vi "MirrorSlidePan.vi"(8 "error in (no error)":errorcluster caption="entrée d'erreur (pas d'erreur)", 11 "ESP301.lvclass":refnum<class "ESP301.lvclass">) -> (0 "error out":errorcluster caption="sortie d'erreur", 3 "ESP301.lvclass Out":refnum<class "ESP301.lvclass">)   [LabVIEW 2019, in "ESP301.lvclass"]
uses:
  ESP301.lvclass
  C:/Programmes Labview/LabscanV1A/DevicesClass/BaseDevice/BaseDevice.lvclass
  ESP301.lvclass/ESP301.ctl
  BaseDevice/ClassQueueMess.ctl
  BaseDevice/Accessor/GetClassEvent.vi
panel:
  out "ESP_pos":refnum<vi>
  out "APDs":bool
  in  "Con/Disc.":bool
  out "Homed":bool
  in  "Enable":bool
  in  "Home":bool caption="MiseAJour"
  out "Moving":bool
  out "Axis Model":string
  out "Valid Ref":bool
  out "BKD Lim":bool
  out "FWD Lim":bool
  in  "Axis 1":u8(ring)=1 items=["1"=1, "2"=2, "3"=3]
  out "ActPos":dbl=60.0 caption="Pos(mm)" min=0.1 step=0.1 format="%#.4f"
  in  "Target":dbl caption="Target(mm)" min=-25000.0 max=25000.0 step=0.0001 format="%#.4f"
  in  "Axis Name":string
  in  "MainProgQ":refnum<queue>
  in  "MainProgQEvent":refnum<user-event>
  in  "Acq":bool
  in  "Stop":bool
  in  "MirrorMotion":u16(ring) caption="MiseAJour" items=["Cam", "APD", "Spectro"]
  out "Init Program":bool
  # "this MUST labeled with class name"
  # "this MUST be present and labeled \"Stop\" and \"Acq\""
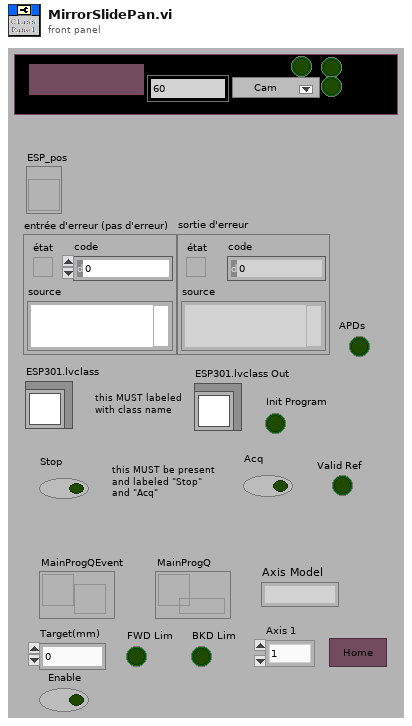
[diagram p1: front panel]
types:
  T1 = cluster{"ESP300mm":refnum<vi>, "ESP300ps":refnum<vi>, "MvgESP300":refnum<vi>}
  T2 = typedef "ClassQueueMess.ctl" = u16
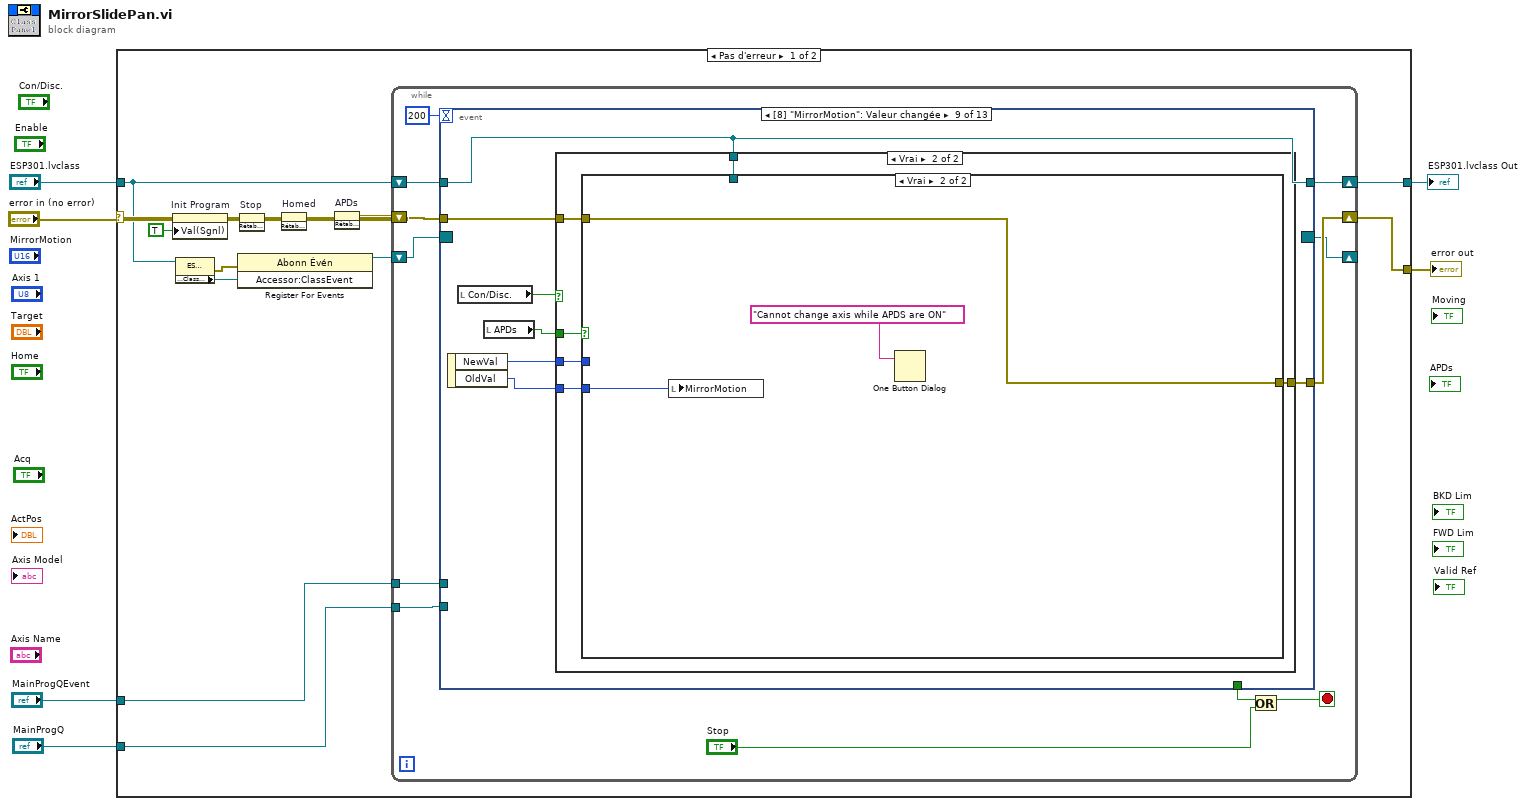
[diagram p0: block diagram]
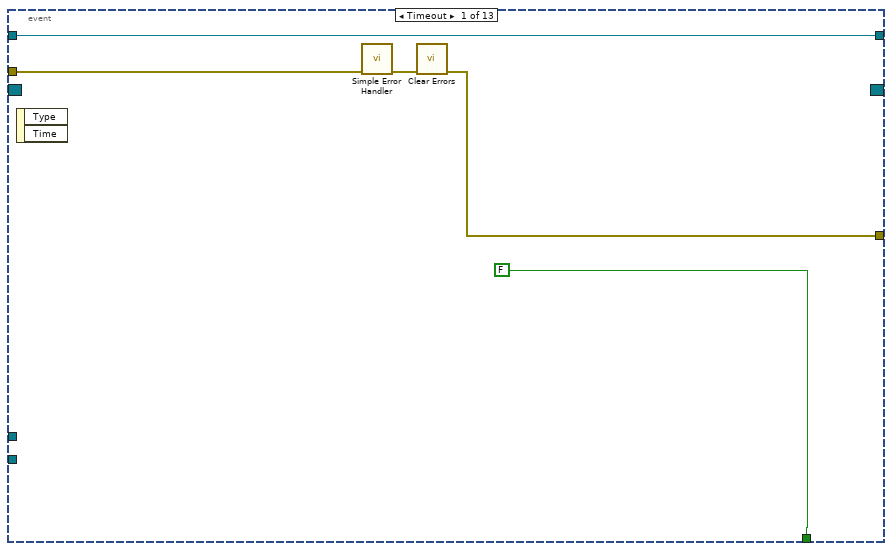
[diagram p2: hidden frame]
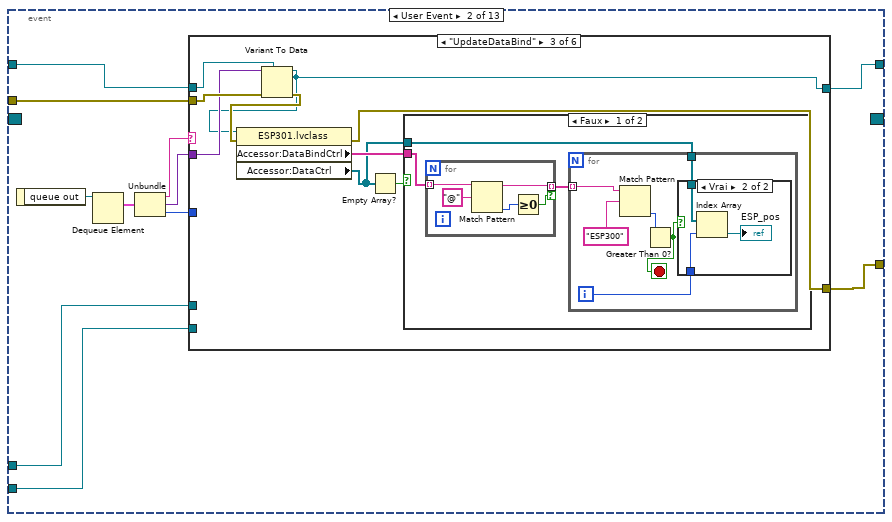
[diagram p3: hidden frame]
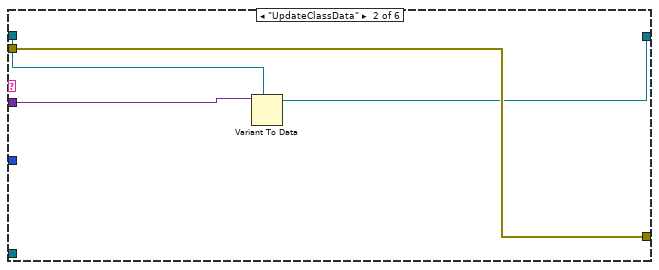
[diagram p5: hidden frame]
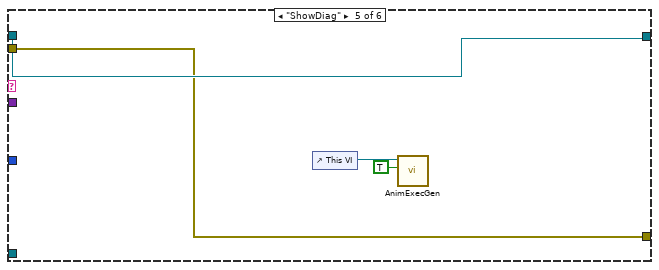
[diagram p9: hidden frame]
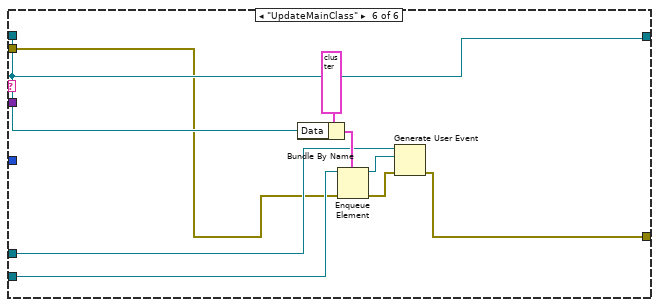
[diagram p10: hidden frame]
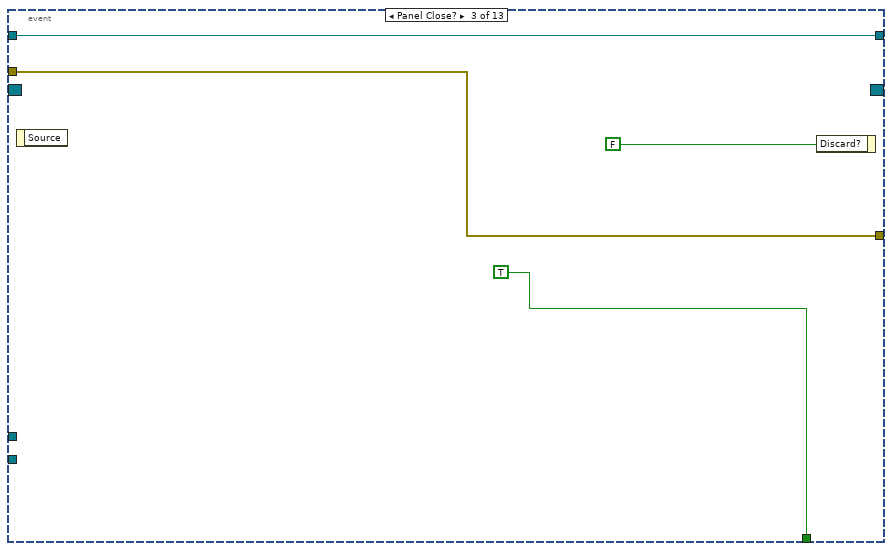
[diagram p11: hidden frame]
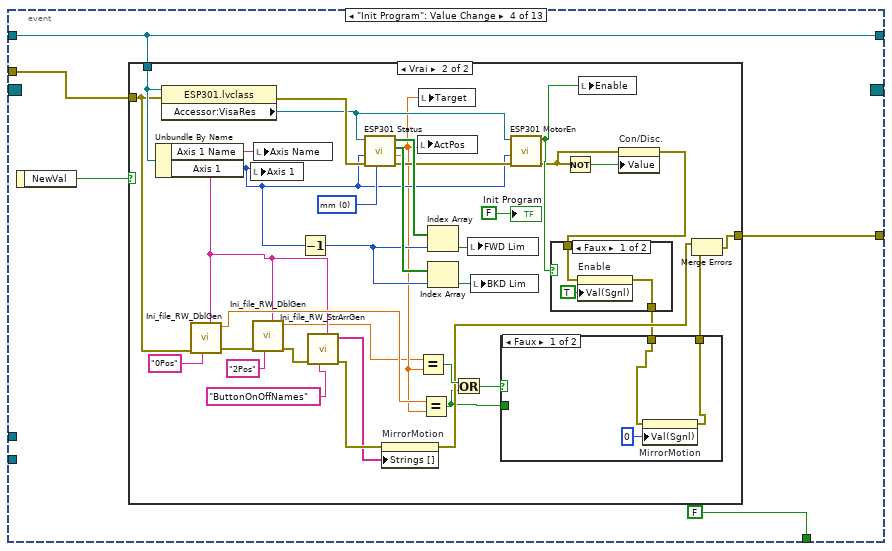
[diagram p12: hidden frame]
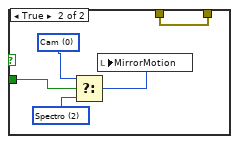
[diagram p15: hidden frame]
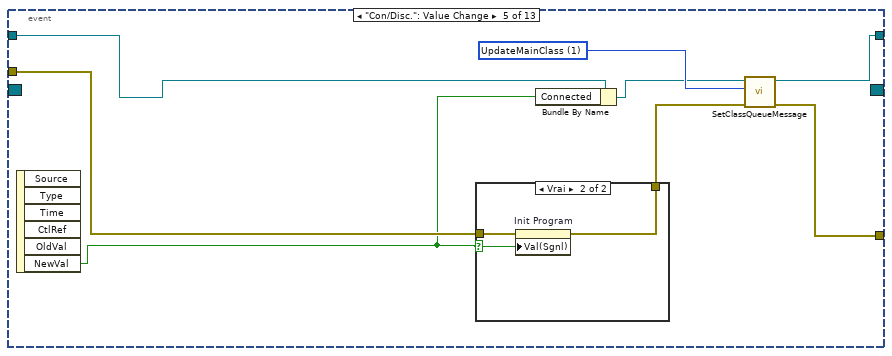
[diagram p16: hidden frame]
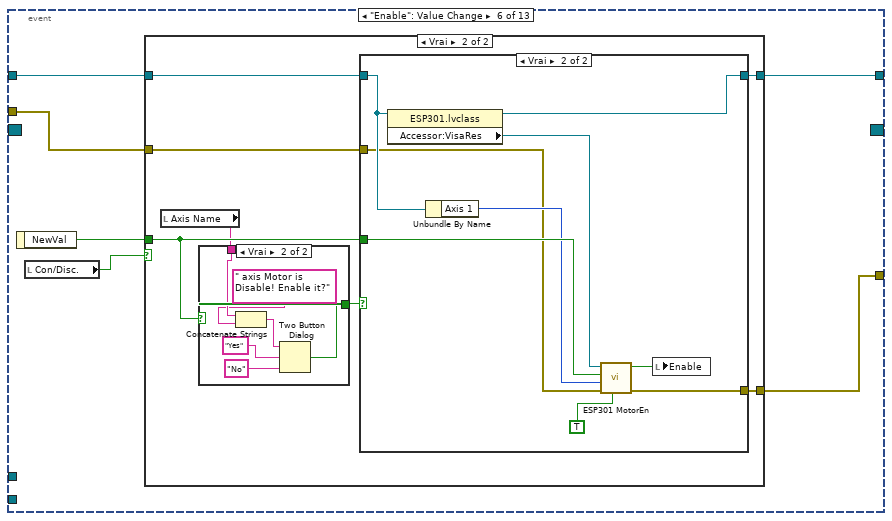
[diagram p18: hidden frame]
diagram:
  n1 = case shown="Pas d'erreur" "error in (no error)" {
    selector: "error in (no error)" -> [w17 w462]
    tunnel: [w20 w462] -> w5
    tunnel: "ESP301.lvclass" -> [w13 w461]
    tunnel: [w18 w461] -> w3
    tunnel: "MainProgQEvent" -> [w11 _]
    tunnel: "MainProgQ" -> [w10 _]
    frame No Error {
      n2 = property on="Init Program" class="Bool (strict)"(error in=w17, "Val(Sgnl)"=TRUE ("Valeur (Signalisation)")) -> (error out=w16:errorcluster)  [unwired: 1 in, 1 out]
      n3 = property class="ESP301.lvclass"(reference=w13) -> (error out=w15:errorcluster, "Accessor:ClassEvent"=w14:refnum<user-event>)  [unwired: 1 in, 1 out]
      n4 = register-events(error in=w15, w14) -> (reference out=w12:refnum<event-registration>)  [unwired: 1 in, 1 out]
      n5 = invoke on="Stop" class="Bool (strict)" method="RétablirValParDéfaut"(error in=w16) -> (error out=w9:errorcluster)  [unwired: 2 in, 2 out]
      n6 = invoke on="Homed" class="Bool (strict)" method="RétablirValParDéfaut"(error in=w9) -> (error out=w8:errorcluster)  [unwired: 2 in, 2 out]
      n7 = invoke on="APDs" class="Bool (strict)" method="RétablirValParDéfaut"(error in=w8) -> (error out=w7:errorcluster)  [unwired: 2 in, 2 out]
      n8 = while {
        shift-right: [w30] -> w20
        shift-left: w7 -> [w31]
        shift-right: [w28] -> w18
        shift-left: w13 -> [w29]
        shift-right: [w26] -> _
        shift-left: w12 -> [w27]
        tunnel: w11 -> [w25]
        tunnel: w10 -> [w24]
        stop <- w22 stop-if-true
        n9 = event shown="[8] \"MirrorMotion\": Valeur changée" {
          selector: w27 -> [_ _ _ _ _ _ _ _ _ _ _ _ _]
          dyn-events: [_ _ _ _ _ _ _ _ _ _ _ _ _] -> w26
          timeout: 200 -> [_ _ _ _ _ _ _ _ _ _ _ _ _]
          tunnel: w31 -> [w35 w47 w97 w103 w156 w167 w207 w225 w259 w320 w383 w397 w419]
          tunnel: [w33 w41 w97 w102 w153 w168 w202 w224 w258 w318 w381 w396 w418] -> w30
          tunnel: w29 -> [w36 w48 w96 w100 w160 w169 w205 w223 w257 w319 w382 w398 w420]
          tunnel: [FALSE _ TRUE FALSE _ _ FALSE _ _ _ _ _ _] -> w23
          tunnel: [w36 w40 w96 w100 w157 w170 w203 w223 w257 w319 w382 w398 w421] -> w28
          tunnel: w25 -> [_ w39 _ _ _ _ _ _ _ _ _ _ _]
          tunnel: w24 -> [_ w38 _ _ _ _ _ _ _ _ _ _ _]
          event Timeout {
            n10 = event-data() -> ()  [unwired: 1 in, 2 out]
            n11 = call <vilib>:"Simple Error Handler.vi"("error in (no error)"=w35) -> ("error out"=w34:errorcluster)  [unwired: 4 in, 4 out]
            n12 = call <vilib>:"Clear Errors.vi"("error in (no error)"=w34) -> ("error out"=w33:errorcluster)  [unwired: 5 in, 1 out]
          }
          event User Event {
            n13 = event-data() -> ("queue out"=w45:refnum<queue>)  [unwired: 1 in]
            n14 = Dequeue Element(queue=w45) -> (element=w46:cluster{"Message":string, "Data":variant, i32})  [unwired: 2 in, 3 out]
            n15 = Unbundle(w46) -> ("Message"=w44:string, "Data"=w43:variant, w42:i32)
            n16 = case shown="\"UpdateDataBind\"" w44 {
              tunnel: w47 -> [w50 w54 w60 w81 w85 w88]
              tunnel: w43 -> [_ w53 w57 _ _ _]
              tunnel: w48 -> [w49 w52 w58 w82 w86 w91]
              tunnel: [w49 w51 w55 w82 w86 w91] -> w40
              tunnel: [w50 w54 w56 w81 w85 w87] -> w41
              tunnel: w42 -> [_ _ _ _ _ _]
              tunnel: w39 -> [_ _ _ _ _ w90]
              tunnel: w38 -> [_ _ _ _ _ w89]
              frame Default {
              }
              frame "UpdateClassData" {
                n17 = Variant To Data(type=w52, Variant=w53) -> (data=w51:refnum<class "ESP301.lvclass">)  [unwired: 1 in, 1 out]
              }
              frame "UpdateDataBind" {
                n18 = Variant To Data(error in=w60, type=w58, Variant=w57) -> (data=w55:refnum<class "ESP301.lvclass">, error out=w59:errorcluster)
                n19 = property class="ESP301.lvclass"(reference=w55, error in=w59) -> (error out=w56:errorcluster, "Accessor:DataBindCtrl"=w62:string[], "Accessor:DataCtrl"=w61:refnum<vi>[])  [unwired: 1 out]
                n20 = Empty Array?(array=w61) -> (empty?=w63:bool)
                n21 = case shown="Faux" w63 {
                  tunnel: w62 -> [w66 _]
                  tunnel: w61 -> [w64 _]
                  frame False {
                    n22 = for {
                      tunnel: w66 -> [w80] mode=indexing
                      tunnel: [w78] -> w65 mode=indexing if=w77
                      n23 = Match Pattern(string=w80, regular expression="@" ("expression régulière")) -> (before substring=w78:string, offset past match=w76:i32)  [unwired: 1 in, 2 out]
                      n24 = Greater Or Equal To 0?(x=w76) -> (x >= 0?=w77:bool)
                    }
                    n25 = for {
                      tunnel: w65 -> [w71] mode=indexing
                      tunnel: w64 -> [w68]
                      i -> [w67]
                      stop <- w69 stop-if-true
                      n26 = Match Pattern(string=w71, regular expression="ESP300" ("nom (aucun)")) -> (offset past match=w70:i32)  [unwired: 1 in, 3 out]
                      n27 = Greater Than 0?(x=w70) -> (x > 0?=w69:bool)
                      n28 = case shown="Vrai" w69 {
                        tunnel: w68 -> [_ w74]
                        tunnel: w67 -> [_ w73]
                        frame False {
                        }
                        frame True {
                          n29 = Index Array(array=w74, index=w73) -> (element=→"ESP_pos":refnum<vi>)
                        }
                      }
                    }
                  }
                  frame True {
                  }
                }
              }
              frame "MeasDone" {
              }
              frame "ShowDiag" {
                n30 = control-ref of="This VI"() -> (w84:refnum<vi>)
                n31 = call <userlib>:"AnimExecGen.vi"("Animer l'exécution ?"=TRUE, "ViRef"=w84) -> ()  [unwired: 9 in, 1 out]
              }
              frame "UpdateMainClass" {
                n32 = Bundle By Name(cluster=cluster{"Message":string, "Data":variant, i32} {"Message"="", "Data"=variant, 0} ("élément"), "Data"=w91) -> (w92:cluster{"Message":string, "Data":variant, i32})
                n33 = Enqueue Element(queue=w89, element=w92, error in (no error)=w88) -> (queue out=w95:refnum<queue>, error out=w94:errorcluster)  [unwired: 1 in, 1 out]
                n34 = Generate User Event(user event=w90, event data cluster=w95, error in=w94) -> (error out=w87:errorcluster)  [unwired: 1 in, 1 out]
              }
            }
          }
          event Panel Close? {
            n35 = event-data() -> ()  [unwired: 1 in, 1 out]
            n36 = event-data("Discard?"=FALSE ("Rejeter ?")) -> ()  [unwired: 1 in, 1 out]
          }
          event "Init Program": Value Change {
            n37 = event-data() -> ("NewVal"=w104:bool)  [unwired: 1 in]
            n38 = case shown="Vrai" w104 {
              tunnel: w103 -> [w105 w127]
              tunnel: [w105 w116] -> w102
              tunnel: w100 -> [_ w139]
              frame False {
              }
              frame True {
                w137 = i8 0 items=["mm", "ps"] ("Input Units")
                n39 = Unbundle By Name(w139) -> ("Axis 1 Name"=w119:string, "Axis 1"=w130:u8)
                n40 = property class="ESP301.lvclass"(reference=w139, error in=w127) -> (error out=w138:errorcluster, "Accessor:VisaRes"=w131:refnum<visa-resource-name>)  [unwired: 1 out]
                n41 = call <userlib>:"Ini_file_RW_DblGen.vi"("Section"=w119, "Key"="0Pos", "Error in"=w127) -> ("Error out"=w125:errorcluster, "ValueOut"=w124:dbl)  [unwired: 6 in]
                n42 = local write "Axis 1"(w130) -> ()
                n43 = call <userlib>:"Ini_file_RW_DblGen.vi"("Section"=w119, "Key"="2Pos", "Error in"=w125) -> ("Error out"=w120:errorcluster, "ValueOut"=w112:dbl)  [unwired: 6 in]
                n44 = local write "Axis Name"(w119) -> ()
                n45 = Decrement(x=w130) -> (x-1=w129:u8)
                n46 = call <userlib>:"Ini_file_RW_StrArrGen.vi"("Section"=w119, "Key"="ButtonOnOffNames", "Error in"=w120) -> ("Error out"=w117:errorcluster, "ValueOut"=w115:string[])  [unwired: 6 in]
                n47 = call <userlib>:"ESP301 Status.vi"("Input Units"=w137, "error in"=w138, "Axis"=w130, "VISA Rsrc"=w131) -> ("error out"=w132:errorcluster, "Position"=w123:dbl, "Low Limit"=w133:bool[], "High Limit"=w134:bool[])  [unwired: 4 in]
                n48 = property on="MirrorMotion" class="MDér (strict)"(error in=w117, "Strings []"=w115) -> (error out=w114:errorcluster)  [unwired: 1 in, 1 out]
                n49 = local write "ActPos"(w123) -> ()
                n50 = Equal?(x=w112, y=w123) -> (x = y?=w122:bool)
                n51 = local write "Target"(w123) -> ()
                n52 = Equal?(x=w124, y=w123) -> (x = y?=w113:bool)
                n53 = Index Array(array=w134, index=w129) -> (element=w135:bool)
                n54 = Index Array(array=w133, index=w129) -> (element=w136:bool)
                n55 = Or(x=w122, y=w113) -> (x .or. y?=w121:bool)
                n56 = local write "FWD Lim"(w135) -> ()
                n57 = local write "BKD Lim"(w136) -> ()
                n58 = call <userlib>:"ESP301 MotorEn.vi"("error in"=w132, "Axis"=w130, "VISA Rsrc"=w131) -> ("error out"=w107:errorcluster, "MotorEnOut"=w111:bool)  [unwired: 7 in]
                n59 = Not(x=w107) -> (.not. x?=w108:bool)
                n60 = local write "Enable"(w111) -> ()
                n61 = property on="Con/Disc." class="Bool (strict)"(error in=w107, "Value"=w108) -> (error out=w106:errorcluster)  [unwired: 1 in, 1 out]
                n62 = case shown="Faux" w111 {
                  tunnel: w106 -> [w143 w144]
                  tunnel: [w142 w144] -> w110
                  frame False {
                    n63 = property on="Enable" class="Bool (strict)"(error in=w143, "Val(Sgnl)"=TRUE ("Valeur (Signalisation)")) -> (error out=w142:errorcluster)  [unwired: 1 in, 1 out]
                  }
                  frame True {
                  }
                }
                n64 = case shown="Faux" w121 {
                  tunnel: w113 -> [_ w152]
                  tunnel: w110 -> [w145 w148]
                  tunnel: [w146 w148] -> w109
                  frame False {
                    n65 = property on="MirrorMotion" class="MDér (strict)"(error in=w145, "Val(Sgnl)"=u16 0 ("Valeur (Signalisation)")) -> (error out=w146:errorcluster)  [unwired: 1 in, 1 out]
                  }
                  frame True {
                    w151 = u16 2 items=["Cam", "APD", "Spectro"] ("MirrorMotion")
                    w150 = u16 0 items=["Cam", "APD", "Spectro"] ("MirrorMotion")
                    n66 = Select(t=w150, s=w152, f=w151) -> (s? t:f=w149:u16)
                    n67 = local write "MirrorMotion"(w149) -> ()
                  }
                }
                n68 = Merge Errors(w114, w109) -> (w116:errorcluster)
                "Init Program" <- FALSE
              }
            }
          }
          event "Con/Disc.": Value Change {
            w159 = T2 1 items=["UpdateClassData", "UpdateMainClass", "UpdateDataBind", "ReInitDevice", "Custom", "ClosePan"] ("Menu déroulant")
            n69 = event-data() -> ("NewVal"=w155:bool)  [unwired: 1 in, 5 out]
            n70 = case shown="Vrai" w155 {
              selector: w155 -> [_ w163]
              tunnel: w156 -> [w161 w164]
              tunnel: [w161 w162] -> w154
              frame False {
              }
              frame True {
                n71 = property on="Init Program" class="Bool (strict)"(error in=w164, "Val(Sgnl)"=w163) -> (error out=w162:errorcluster)  [unwired: 1 in, 1 out]
              }
            }
            n72 = Bundle By Name(cluster=w160, "Connected"=w155) -> (w158:refnum<class "ESP301.lvclass">)
            n73 = call-dynamic "SetClassQueueMessage.vi"("ErrorIn(No Error)"=w154, "Menu déroulant"=w159, "DefaultDev.lvclass"=w158) -> ("sortie d'erreur"=w153:errorcluster, "DefaultDev.lvclass Out"=w157:refnum<class "ESP301.lvclass">)  [unwired: 7 in]
          }
          event "Enable": Value Change {
            n74 = event-data() -> ("NewVal"=w166:bool)  [unwired: 1 in]
            n75 = local read "Con/Disc."() -> (w165:bool)
            n76 = case shown="Vrai" w165 {
              tunnel: [w172 w179] -> w170
              tunnel: w169 -> [w172 w178]
              tunnel: [w171 w177] -> w168
              tunnel: w167 -> [w171 w176]
              tunnel: w166 -> [_ w174]
              frame False {
              }
              frame True {
                n77 = local read "Axis Name"() -> (w173:string)
                n78 = case shown="Vrai" w174 {
                  selector: w174 -> [w180 _]
                  tunnel: [w180 w184] -> w175
                  tunnel: w173 -> [_ w183]
                  frame False {
                  }
                  frame True {
                    n79 = Concatenate Strings(w183, " axis Motor is Disable! Enable it?" ("message")) -> (w181:string)
                    n80 = Two Button Dialog(message=w181, 1:"No" ("Nom du bouton F (\"Annuler\")"), 2:"Yes" ("Nom du bouton V (\"OK\")")) -> (T button?=w184:bool)
                  }
                }
                n81 = case shown="Vrai" w175 {
                  tunnel: w174 -> [_ w194]
                  tunnel: [w187 w193] -> w179
                  tunnel: w178 -> [w187 w192]
                  tunnel: [w188 w190] -> w177
                  tunnel: w176 -> [w188 w189]
                  frame False {
                  }
                  frame True {
                    n82 = property class="ESP301.lvclass"(reference=w192) -> (reference out=w193:refnum<class "ESP301.lvclass">, "Accessor:VisaRes"=w196:refnum<visa-resource-name>)  [unwired: 1 in, 1 out]
                    n83 = Unbundle By Name(w192) -> ("Axis 1"=w191:u8)
                    n84 = call <userlib>:"ESP301 MotorEn.vi"("Set"=TRUE, "error in"=w189, "Axis"=w191, "MotorEn"=w194, "VISA Rsrc"=w196) -> ("error out"=w190:errorcluster, "MotorEnOut"=w197:bool)  [unwired: 5 in]
                    n85 = local write "Enable"(w197) -> ()
                  }
                }
              }
            }
          }
          event "Axis 1": Value Change {
            w201 = T2 1 items=["UpdateClassData", "UpdateMainClass", "UpdateDataBind", "ReInitDevice", "Custom", "ClosePan"] ("Menu déroulant")
            n86 = event-data() -> ("NewVal"=w198:u8)  [unwired: 1 in]
            n87 = local read "Con/Disc."() -> (w199:bool)
            n88 = case shown="Vrai" w199 {
              tunnel: w207 -> [w208 w221]
              tunnel: w205 -> [_ w220]
              tunnel: [w208 w217] -> w200
              tunnel: w198 -> [_ w211]
              frame False {
              }
              frame True {
                w216 = i8 0 items=["mm", "ps"] ("Input Units")
                n89 = property class="ESP301.lvclass"(reference=w220, error in=w221) -> (error out=w218:errorcluster, "Accessor:VisaRes"=w219:refnum<visa-resource-name>)  [unwired: 1 out]
                n90 = local write "Axis 1"(w211) -> ()
                n91 = Decrement(x=w211) -> (x-1=w210:u8)
                n92 = call <userlib>:"ESP301 Status.vi"("Input Units"=w216, "error in"=w218, "Axis"=w211, "VISA Rsrc"=w219) -> ("error out"=w217:errorcluster, "Position"=w209:dbl, "Low Limit"=w212:bool[], "High Limit"=w215:bool[])  [unwired: 4 in]
                n93 = Index Array(array=w215, index=w210) -> (element=w213:bool)
                n94 = Index Array(array=w212, index=w210) -> (element=w214:bool)
                n95 = local write "Target"(w209) -> ()
                n96 = local write "ActPos"(w209) -> ()
                n97 = local write "FWD Lim"(w213) -> ()
                n98 = local write "BKD Lim"(w214) -> ()
              }
            }
            n99 = Bundle By Name(cluster=w205, "Axis 1"=w198) -> (w204:refnum<class "ESP301.lvclass">)
            n100 = call-dynamic "SetClassQueueMessage.vi"("ErrorIn(No Error)"=w200, "Menu déroulant"=w201, "DefaultDev.lvclass"=w204) -> ("sortie d'erreur"=w202:errorcluster, "DefaultDev.lvclass Out"=w203:refnum<class "ESP301.lvclass">)  [unwired: 7 in]
          }
          event "Home": Value Change {
            n101 = event-data() -> ("NewVal"=w226:bool)  [unwired: 1 in]
            n102 = local read "Con/Disc."() -> (w222:bool)
            n103 = case shown="Vrai" w222 {
              tunnel: w226 -> [_ w232]
              tunnel: w223 -> [_ w231]
              tunnel: w225 -> [w227 w230]
              tunnel: [w227 w229] -> w224
              frame False {
              }
              frame True {
                n104 = local read "APDs"() -> (w228:bool)
                n105 = case shown="Faux" w228 {
                  tunnel: w232 -> [w236 _]
                  tunnel: w231 -> [w235 _]
                  tunnel: w230 -> [w234 w252]
                  tunnel: [w233 w252] -> w229
                  frame False {
                    n106 = case shown="Vrai" w236 {
                      tunnel: w235 -> [_ w251]
                      tunnel: w234 -> [w237 w243]
                      tunnel: [w237 w241] -> w233
                      frame False {
                      }
                      frame True {
                        w247 = i8 0 items=["mm", "ps"] ("Input Units")
                        n107 = property class="ESP301.lvclass"(reference=w251, error in=w243) -> (error out=w249:errorcluster, "Accessor:VisaRes"=w250:refnum<visa-resource-name>)  [unwired: 1 out]
                        n108 = control-ref of="Moving"() -> (w242:refnum<vi>)
                        n109 = control-ref of="ActPos"() -> (w245:refnum<vi>)
                        n110 = local read "Axis 1"() -> (w248:u8)
                        n111 = Bundle By Name(cluster=T1 {"ESP300mm"=refnum, "ESP300ps"=refnum, "MvgESP300"=refnum} ("ESP301Ref"), "ESP300mm"=w245, "MvgESP300"=w242) -> (w244:T1)
                        n112 = call <userlib>:"Wait_At_Wire_Bool.vi"("Wait (ms)"=u32 250, "error in (no error)"=FALSE) -> ("error out"=w240:bool)  [unwired: 7 in, 2 out]
                        n113 = local write "Home"(w240) -> ()
                        n114 = call <userlib>:"ESP301 Home.vi"("Input Units"=w247, "ESP301Ref"=w244, "error in"=w249, "Axis"=w248, "VISA Rsrc"=w250) -> ("error out"=w241:errorcluster)  [unwired: 6 in]
                      }
                    }
                  }
                  frame True {
                    n115 = One Button Dialog(message="Cannot change axis while APDS are ON") -> ()  [unwired: 1 in, 1 out]
                  }
                }
              }
            }
          }
          event "MirrorMotion": Value Change {
            n116 = event-data() -> ("NewVal"=w260:u16, "OldVal"=w254:u16)  [unwired: 1 in]
            n117 = local read "Con/Disc."() -> (w256:bool)
            n118 = local read "APDs"() -> (w255:bool)
            n119 = case shown="Vrai" w256 {
              tunnel: w260 -> [_ w267]
              tunnel: w259 -> [w261 w266]
              tunnel: [w261 w265] -> w258
              tunnel: w257 -> [_ w264]
              tunnel: w255 -> [_ w263]
              tunnel: w254 -> [_ w262]
              frame False {
              }
              frame True {
                n120 = case shown="Vrai" w263 {
                  tunnel: w267 -> [w271 _]
                  tunnel: w266 -> [w272 w316]
                  tunnel: [w270 w316] -> w265
                  tunnel: w264 -> [w275 _]
                  tunnel: w262 -> [_ w314]
                  frame False {
                    n121 = local read "Axis Name"() -> (w276:string)
                    n122 = local read "ESP_pos"() -> (w273:refnum<vi>)
                    n123 = Not A Number/Path/Refnum?(number/path/refnum=w273) -> (NaN/Path/Refnum?=w274:bool)
                    n124 = case shown="0, Par défaut" w271 {
                      tunnel: w272 -> [w283 w305 w311]
                      tunnel: [w282 w307 w313] -> w268
                      tunnel: w275 -> [w290 _ _]
                      tunnel: w276 -> [w284 w302 w308]
                      frame 0, Default {
                        w291 = i8 0 items=["mm", "ps"] ("Input Units")
                        # "Cam"
                        n125 = property class="ESP301.lvclass"(reference=w290, error in=w283) -> (error out=w300:errorcluster, "Accessor:VisaRes"=w301:refnum<visa-resource-name>)  [unwired: 1 out]
                        n126 = control-ref of="Moving"() -> (w296:refnum<vi>)
                        n127 = control-ref of="ActPos"() -> (w298:refnum<vi>)
                        n128 = local read "Axis 1"() -> (w299:u8)
                        n129 = Bundle By Name(cluster=T1 {"ESP300mm"=refnum, "ESP300ps"=refnum, "MvgESP300"=refnum} ("ESP301Ref"), "ESP300mm"=w298, "MvgESP300"=w296) -> (w297:T1)
                        n130 = call <userlib>:"ESP301 Home.vi"("Input Units"=w291, "ESP301Ref"=w297, "error in"=w300, "Axis"=w299, "VISA Rsrc"=w301) -> ("error out"=w288:errorcluster)  [unwired: 6 in]
                        n131 = call <userlib>:"Wait_At_Wire_Bool.vi"("Wait (ms)"=u32 250, "error in (no error)"=FALSE) -> ("error out"=w295:bool)  [unwired: 7 in, 2 out]
                        n132 = call <userlib>:"Ini_file_RW_DblGen.vi"("Section"=w284, "Key"="0Pos", "Error in"=w288) -> ("Error out"=w287:errorcluster, "ValueOut"=w286:dbl)  [unwired: 6 in]
                        n133 = local write "Home"(w295) -> ()
                        n134 = property on="Target" class="NumNb (strict)"(error in=w287, "Val(Sgnl)"=w286) -> (error out=w282:errorcluster)  [unwired: 1 in, 1 out]
                        "Homed" <- TRUE ("Homed")
                      }
                      frame 1 {
                        # "APD"
                        n135 = call <userlib>:"Ini_file_RW_DblGen.vi"("Section"=w302, "Key"="1Pos", "Error in"=w305) -> ("Error out"=w304:errorcluster, "ValueOut"=w306:dbl)  [unwired: 6 in]
                        n136 = property on="Target" class="NumNb (strict)"(error in=w304, "Val(Sgnl)"=w306) -> (error out=w307:errorcluster)  [unwired: 1 in, 1 out]
                      }
                      frame 2 {
                        # "Spectro"
                        n137 = call <userlib>:"Ini_file_RW_DblGen.vi"("Section"=w308, "Key"="2Pos", "Error in"=w311) -> ("Error out"=w310:errorcluster, "ValueOut"=w312:dbl)  [unwired: 6 in]
                        n138 = property on="Target" class="NumNb (strict)"(error in=w310, "Val(Sgnl)"=w312) -> (error out=w313:errorcluster)  [unwired: 1 in, 1 out]
                      }
                    }
                    n139 = case shown="Faux" w274 {
                      tunnel: w273 -> [w280 _]
                      tunnel: w271 -> [w279 _]
                      tunnel: w272 -> [w278 w281]
                      tunnel: [w277 w281] -> w269
                      frame False {
                        n140 = property class="Cmde"(reference=w280, error in=w278, "Val(Sgnl)"=w279) -> (error out=w277:errorcluster)  [unwired: 1 out]
                      }
                      frame True {
                      }
                    }
                    n141 = Merge Errors(w268, w269) -> (w270:errorcluster)
                  }
                  frame True {
                    n142 = local write "MirrorMotion"(w314) -> ()
                    n143 = One Button Dialog(message="Cannot change axis while APDS are ON") -> ()  [unwired: 1 in, 1 out]
                  }
                }
              }
            }
          }
          event "MirrorMotion": Shortcut Menu Selection (User) {
            n144 = event-data() -> ("ItemTag"=w321:string)  [unwired: 1 in]
            n145 = local read "Axis Name"() -> (w317:string)
            n146 = case shown="Par défaut" w321 {
              tunnel: w320 -> [w322 w328 w341 w344 w359 w371]
              tunnel: [w322 w330 w341 w347 w358 w370] -> w318
              tunnel: w317 -> [_ w329 _ w345 w356 w368]
              frame Default {
              }
              frame "ElementsNames" {
                n147 = call "Set Button Elements Text"("error in (no error)"=w328) -> ("Button 2 Text"=w323:string, "Button 1 Text"=w324:string, "Button 0 Text"=w325:string, "Save"=w326:bool, "error out"=w327:errorcluster)  [unwired: 14 in]
                n148 = case shown="Vrai" w326 {
                  tunnel: w327 -> [w331 w338]
                  tunnel: [w331 w337] -> w330
                  tunnel: w329 -> [_ w336]
                  tunnel: w325 -> [_ w335]
                  tunnel: w324 -> [_ w334]
                  tunnel: w323 -> [_ w332]
                  frame False {
                  }
                  frame True {
                    n149 = Build Array(w335, w334, w332) -> (w333:string[])
                    n150 = property on="MirrorMotion" class="MDér (strict)"("Strings []"=w333) -> ()  [unwired: 2 in, 2 out]
                    n151 = call <userlib>:"Ini_file_RW_StrArrGen.vi"("Section"=w336, "Key"="ButtonOnOffNames", "Error in"=w338, "Write"=TRUE, "ValueIn"=w333) -> ("Error out"=w337:errorcluster)  [unwired: 4 in, 1 out]
                  }
                }
              }
              frame "SetAPDCheckOff" {
                n152 = local write "APDs"(FALSE ("APDs")) -> ()
              }
              frame "0 Position" {
                n153 = call "Set Element 0 Position"("error in (no error)"=w344) -> ("Element 0 Position(mm)"=w348:dbl, "Save"=w346:bool, "error out"=w343:errorcluster)  [unwired: 16 in]
                n154 = case shown="Vrai" w346 {
                  tunnel: w348 -> [_ w355]
                  tunnel: w343 -> [w349 w352]
                  tunnel: [w349 w351] -> w347
                  tunnel: w345 -> [_ w350]
                  frame False {
                  }
                  frame True {
                    n155 = call <userlib>:"Ini_file_RW_DblGen.vi"("Section"=w350, "Key"="0Pos", "Error in"=w352, "Write"=TRUE, "ValueIn"=w355) -> ("Error out"=w351:errorcluster)  [unwired: 4 in, 1 out]
                  }
                }
              }
              frame "1 Position" {
                n156 = call "Set Element 1 Position"() -> ("Element 1 Position(mm)"=w360:dbl, "Save"=w357:bool)  [unwired: 17 in, 1 out]
                n157 = case shown="Vrai" w357 {
                  tunnel: w360 -> [_ w367]
                  tunnel: w359 -> [w361 w364]
                  tunnel: [w361 w363] -> w358
                  tunnel: w356 -> [_ w362]
                  frame False {
                  }
                  frame True {
                    n158 = call <userlib>:"Ini_file_RW_DblGen.vi"("Section"=w362, "Key"="1Pos", "Error in"=w364, "Write"=TRUE, "ValueIn"=w367) -> ("Error out"=w363:errorcluster)  [unwired: 4 in, 1 out]
                  }
                }
              }
              frame "2 Position" {
                n159 = call "Set Element 2 Position"() -> ("Element 2 Position(mm)"=w372:dbl, "Save"=w369:bool)  [unwired: 17 in, 1 out]
                n160 = case shown="Vrai" w369 {
                  tunnel: w372 -> [_ w379]
                  tunnel: w371 -> [w373 w376]
                  tunnel: [w373 w375] -> w370
                  tunnel: w368 -> [_ w374]
                  frame False {
                  }
                  frame True {
                    n161 = call <userlib>:"Ini_file_RW_DblGen.vi"("Section"=w374, "Key"="2Pos", "Error in"=w376, "Write"=TRUE, "ValueIn"=w379) -> ("Error out"=w375:errorcluster)  [unwired: 4 in, 1 out]
                  }
                }
              }
            }
          }
          event "ActPos": Shortcut Menu Selection (User) {
            n162 = event-data() -> ("ItemTag"=w384:string)  [unwired: 1 in]
            n163 = local read "Axis Name"() -> (w380:string)
            n164 = case shown="\"Goto\"" w384 {
              tunnel: w383 -> [w385 w389]
              tunnel: [w385 w388] -> w381
              tunnel: w380 -> [_ w386]
              frame Default {
              }
              frame "Goto" {
                n165 = call "Go to Position"() -> ("Target Position(mm)"=w390:dbl, "Goto"=w387:bool)  [unwired: 17 in, 1 out]
                n166 = case shown="Vrai" w387 {
                  tunnel: w390 -> [_ w392]
                  tunnel: w389 -> [w391 w393]
                  tunnel: [w391 w393] -> w388
                  tunnel: w386 -> [_ _]
                  frame False {
                  }
                  frame True {
                    n167 = property on="Target" class="NumNb (strict)"("Val(Sgnl)"=w392) -> ()  [unwired: 2 in, 2 out]
                  }
                }
              }
            }
          }
          event "Target": Value Change {
            n168 = event-data() -> ("NewVal"=w395:dbl)  [unwired: 1 in]
            n169 = local read "Con/Disc."() -> (w394:bool)
            n170 = case shown="Vrai" w394 {
              tunnel: w398 -> [_ w415]
              tunnel: w397 -> [w399 w414]
              tunnel: [w399 w407] -> w396
              tunnel: w395 -> [_ w406]
              frame False {
              }
              frame True {
                w408 = i8 0 items=["mm", "ps"] ("Input Units")
                n171 = property class="ESP301.lvclass"(reference=w415, error in=w414) -> (error out=w410:errorcluster, "Accessor:VisaRes"=w411:refnum<visa-resource-name>)  [unwired: 1 out]
                n172 = control-ref of="Moving"() -> (w412:refnum<vi>)
                n173 = control-ref of="ActPos"() -> (w413:refnum<vi>)
                n174 = local read "Axis 1"() -> (w409:u8)
                n175 = Bundle By Name(cluster=T1 {"ESP300mm"=refnum, "ESP300ps"=refnum, "MvgESP300"=refnum} ("ESP301Ref"), "ESP300mm"=w413, "MvgESP300"=w412) -> (w401:T1)
                n176 = call <userlib>:"ESP301 Goto.vi"("Input Units"=w408, "ESP301Ref"=w401, "error in"=w410, "Axis"=w409, "Position"=w406, "VISA Rsrc"=w411) -> ("error out"=w407:errorcluster, "HighLim"=w403:bool, "Pos Out"=w405:dbl, "Warning"=w402:bool, "LowLim"=w404:bool)  [unwired: 1 in]
                n177 = local write "ActPos"(w405) -> ()
                n178 = case shown="Vrai" w402 {
                  tunnel: w404 -> [_ w417]
                  tunnel: w403 -> [_ w416]
                  frame False {
                  }
                  frame True {
                    n179 = local write "FWD Lim"(w416) -> ()
                    n180 = local write "BKD Lim"(w417) -> ()
                  }
                }
              }
            }
          }
          event "Axis Name": Shortcut Menu Selection (User) {
            n181 = event-data() -> ("ItemTag"=w422:string)  [unwired: 1 in]
            n182 = case shown="\"ChangeName\"" w422 {
              tunnel: [w424 w428 w439 w443 w448] -> w421
              tunnel: w420 -> [w424 w428 w439 w443 w449]
              tunnel: w419 -> [w423 w427 w437 w441 w450]
              tunnel: [w423 w425 w436 w440 w445] -> w418
              frame Default {
              }
              frame "Change Axis" {
                n183 = call "Set Mirror Axis"("error in (no error)"=w427) -> ("Mirror Axis"=w430:dbl, "Save"=w429:bool, "error out"=w426:errorcluster)  [unwired: 16 in]
                n184 = case shown="Vrai" w429 {
                  tunnel: w426 -> [w431 w435]
                  tunnel: [w431 w434] -> w425
                  tunnel: w430 -> [_ w433]
                  frame False {
                  }
                  frame True {
                    n185 = To Unsigned Byte Integer(number=w433) -> (unsigned 8bit integer=w432:u8)
                    n186 = property on="Axis 1" class="MDér (strict)"(error in=w435, "Val(Sgnl)"=w432) -> (error out=w434:errorcluster)  [unwired: 1 in, 1 out]
                  }
                }
              }
              frame "Home Axis" {
                n187 = property on="Home" class="Bool (strict)"(error in=w437, "Val(Sgnl)"=TRUE ("Valeur (Signalisation)")) -> (error out=w436:errorcluster)  [unwired: 1 in, 1 out]
              }
              frame "EnableAxis" {
                n188 = property on="Enable" class="Bool (strict)"(error in=w441, "Val(Sgnl)"=TRUE ("Valeur (Signalisation)")) -> (error out=w440:errorcluster)  [unwired: 1 in, 1 out]
              }
              frame "ChangeName" {
                n189 = call "SaveAxisName"("Enable"=TRUE, "error in (no error)"=w450) -> ("Name"=w444:string, "Save"=w447:bool, "error out"=w446:errorcluster)  [unwired: 15 in]
                n190 = case shown="Vrai" w447 {
                  tunnel: w449 -> [w453 w460]
                  tunnel: [w453 w458] -> w448
                  tunnel: w446 -> [w452 w457]
                  tunnel: [w452 w456] -> w445
                  tunnel: w444 -> [_ w455]
                  frame False {
                  }
                  frame True {
                    w454 = T2 1 items=["UpdateClassData", "UpdateMainClass", "UpdateDataBind", "ReInitDevice", "Custom", "ClosePan"] ("Menu déroulant")
                    n191 = Bundle By Name(cluster=w460, "Axis 1 Name"=w455) -> (w459:refnum<class "ESP301.lvclass">)
                    n192 = local write "Axis Name"(w455) -> ()
                    n193 = call-dynamic "SetClassQueueMessage.vi"("ErrorIn(No Error)"=w457, "Menu déroulant"=w454, "DefaultDev.lvclass"=w459) -> ("sortie d'erreur"=w456:errorcluster, "DefaultDev.lvclass Out"=w458:refnum<class "ESP301.lvclass">)  [unwired: 7 in]
                  }
                }
              }
            }
          }
        }
        n194 = Or(x=w23, y="Stop") -> (x .or. y?=w22:bool)
      }
    }
    frame Error {
    }
  }
  "error out" <- w5
  "ESP301.lvclass Out" <- w3
